vi "GetNewStepOutRowNum.vi"(8 "lastStat":enum16{"section", "step"}(ring), 11 "lastRowNum":i32) -> (3 "outRowNum":i32)   [LabVIEW 2010]
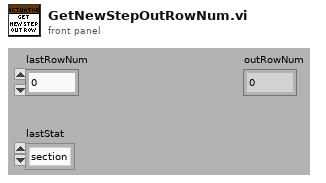
[diagram p1: front panel]
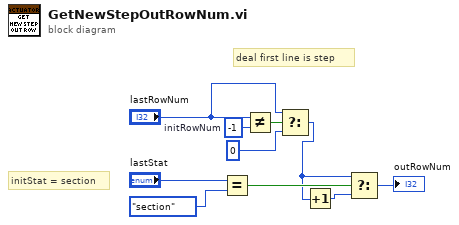
[diagram p0: block diagram]
diagram:
  w8 = -1  # initRowNum
  # "initStat = section"
  # "deal first line is step"
  n1 = Equal?(x="lastStat", y=enum16{"section", "step"}."section") -> (x = y?=w10:bool)
  n2 = Not Equal?(x="lastRowNum", y=w8) -> (x != y?=w7:bool)
  n3 = Select(t="lastRowNum", s=w7, f=0) -> (s? t:f=w5:i32)
  n4 = Increment(x=w5) -> (x+1=w9:i32)
  n5 = Select(t=w5, s=w10, f=w9) -> (s? t:f=→"outRowNum":i32)
